vi "WaitForBufferExample.vi"() -> ()   [LabVIEW 2012]
doc: "A short program to demonstrate the fundamentals of control and image acquision with the pco.camera series. The program records a sequence of images, with \"live\" updating, until the \"StopRecording\" button is pressed. A subset of recorded images is then read out from the camera RAM. Warning: Limit the number of images read back tfrom the camera RAM to a reasonable number. Images are stored as a three-dimensional array, which can very large. Use ctrl-H for more help on the individual controls and indicators.\n\nCopyright 2004, the Cooke Corporation."
panel:
  out "bClose":bool
  in  "Quit":bool
  in  "ImageNr":i32
  in  "Image":i32
  out "BufNr1":i16
  out "BufNr0":i16
  in  "bUseBuffer1":bool
  in  "bUseBuffer0":bool
  in  "ROIX1":u16=1 min=1
  in  "ROIY1":u16=1 min=1
  in  "ROIY0":u16=1 min=1
  in  "ROIX0":u16=1 min=1
  in  "InterfaceType":u16(ring)=5 items=["IEEE1394 - Firewire", "IEEE1394/Firewire", "Matrox Helios Camera Link", "Silicon Software ME3 Camera Link", "National Instruments Camera Link", "Gigabit Ethernet", "USB", "Reserved", "Reserved", "Reserved", "Generic Camera Link with CLSER.DLL"]
  out "Bits/pixel":u16
  in  "Readout":bool
  in  "Record":bool
  in  "Open StructureIn":T1={"Size"=88, "InterfaceType"=0, "Camera Number"=0, "CameraNumAtInterface"=0, "OpenFlags"=[], "OpenDWFlags"=[], "OpenPtrs"=[]}
  in  "Stop":u32=10 min=1
  in  "Start":u32=1 min=1
  in  "DelayTimeBase":u16(ring)=2 items=["nanoseconds", "microseconds", "milliseconds"]
  in  "ExposureTimeBase":u16(ring)=2 items=["nanoseconds", "microseconds", "milliseconds"]
  in  "Exposure":u32=10
  in  "Delay":u32
  out "Reading":bool
  in  "StorageMode":bool
  out "ImageCount":u32
  in  "Rate":i32
  out "Image":u16[][](graph)
  in  "TriggerMode":u16(ring) items=["Auto", "Software", "External sequence start ", "External exposure control"]
  # "A short program to demonstrate the fundamentals of control and image acquision with the pco.camera series. The program records a sequence of images, with \"live\" updating, until the \"StopRecording\" button is pressed. A subset of recorded images is then read out from the camera RAM. WARNING: Limit the number of images read back tfrom the camera RAM to a reasonable number. Images are stored as a three-dimensional array, which can very large.  Use ctrl-H for more help on the individual controls and indicators."
  # "pco.labview"
  # "1) Setup camera:"
  # "FIFO"
  # "Recorder"
  # "2) Record  images:"
  # "3) Read out images:"
  # "4) Display image:"
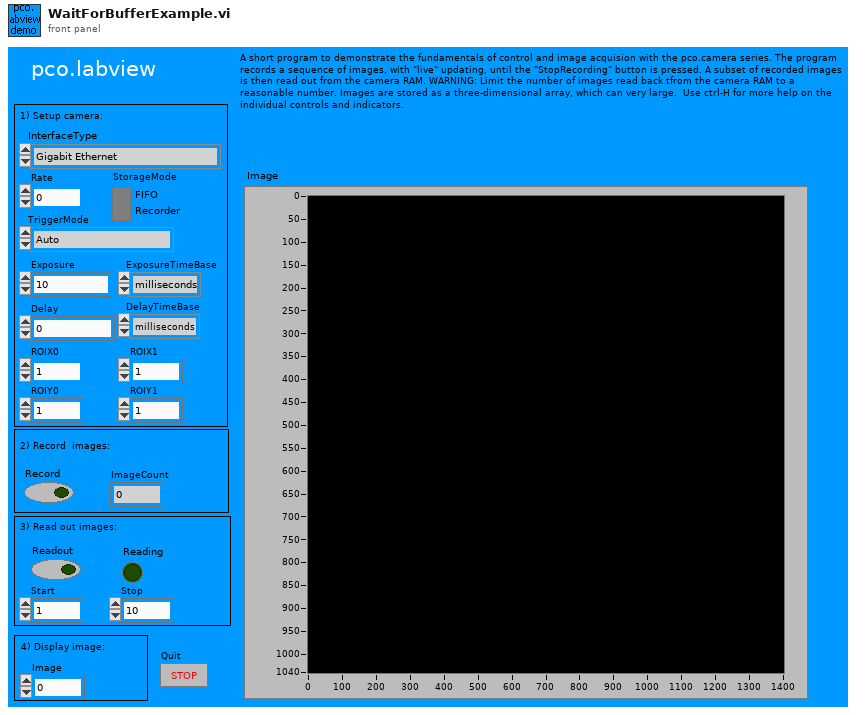
[diagram p1: front panel]
types:
  T1 = cluster{"Size":u16, "InterfaceType":u16, "Camera Number":u16, "CameraNumAtInterface":u16, "OpenFlags":u16[], "OpenDWFlags":u32[], "OpenPtrs":u32[]}
  T2 = cluster{"Size":u16, "CamType":u16, "CamSubType":u16, "SerialNumber":u32, "HWVersion":u32, "FWVersion":u32, "InterfaceType":u16, "HardwareVersion":cluster{"BoardNum":u16, "HWVersions":cluster{"BoardName":string, "BatchNumber":u16, "MinorRevision":u8, "MajorRevision":u8, "Variant":u16}[]}, "FirmwareVersion":cluster{"DeviceNum":u16, "FWVersions":cluster{"DeviceName":string, "MinorRevision":u8, "MajorRevision":u8, "Variant":u16}[]}}
  T3 = cluster{"Size":u16, "SensorTypeDESC":u16, "SensorSubtypeDESC":u16, "MaxHorizontalResStdDESC":u16, "MaxVerticalResStdDESC":u16, "MaxHorizontalResExtDESC":u16, "MaxVerticalResExtDESC":u16, "DynResDESC":u16, "MaxBinHorzDESC":u16, "BinHorzStepDESC":bool, "MaxBinVertDESC":u16, "BinVertStepDESC":bool, "ROIHorzStepDESC":u16, "ROIVertStepDESC":u16, "NumADCDESC":u16, "IRDESC":bool, "MinDelayDESC":u32, "MaxDelayDESC":u32, "MinDelayStepDESC":u32, "MinExpoDESC":u32, "MaxExpoDESC":u32, "MinExpoStepDESC":u32, "MinDelayIRDESC":u32, "MaxDelayIRDESC":u32, "MinExpoIRDESC":u32, "MaxExpoIRDESC":u32, "TimeTableDESC":bool, "DoubleImageDESC":bool, "MinCoolSetDESC":i16, "MaxCoolSetDESC":i16, "MDefaultCoolSetDESC":i16, "PowerDownModeDESC":bool, "OffsetRegDESC":bool, "ColorPattern":cluster{"UpperLeftColor":u8, "UpperRightColor":u8, "LowerLeftColor":u8, "LowerRightColor":u8}, "PatternTypeDESC":bool, "PixelRates":u32[], "CoversionFactors":u16[], "Reserved":u32[], "NoiseFilterCapable":bool, "HotPixelCapable":bool, "HotPixelWithNoiseFilter":bool, "ASCIITimeCapable":bool, "Extended Description":bool, "Get Extended":bool, "Reserved Flag 1":bool, "Reserved Flag 2":bool}
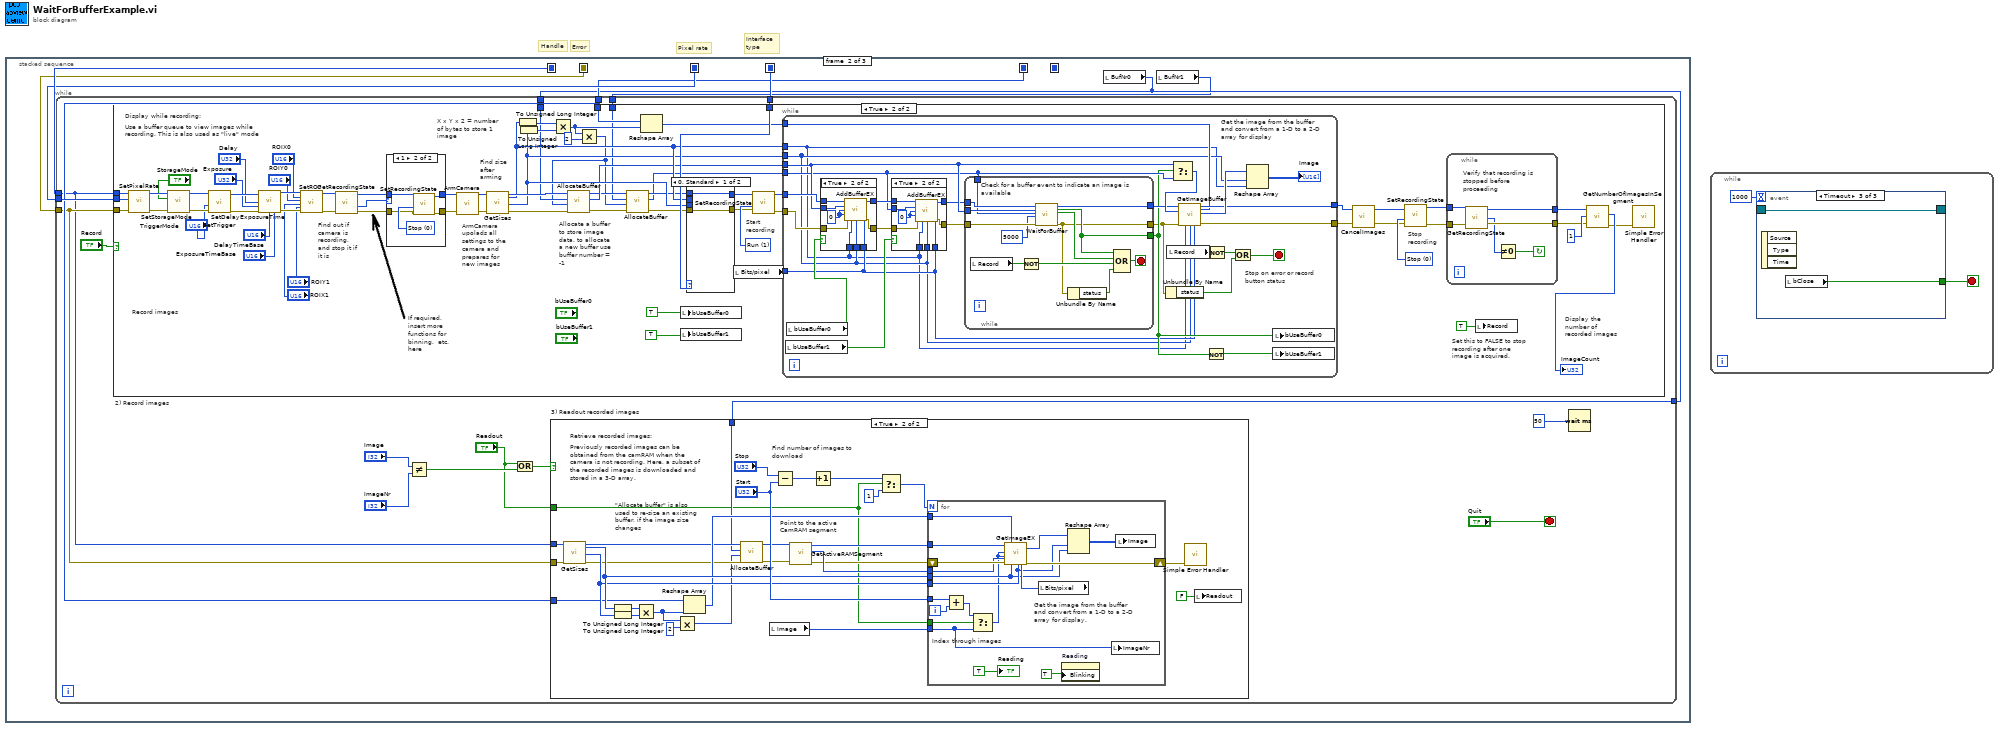
[diagram p0: block diagram]
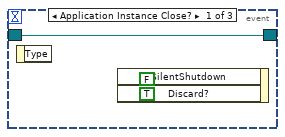
[diagram p2: hidden frame]
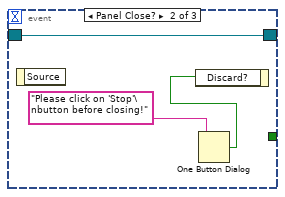
[diagram p3: hidden frame]
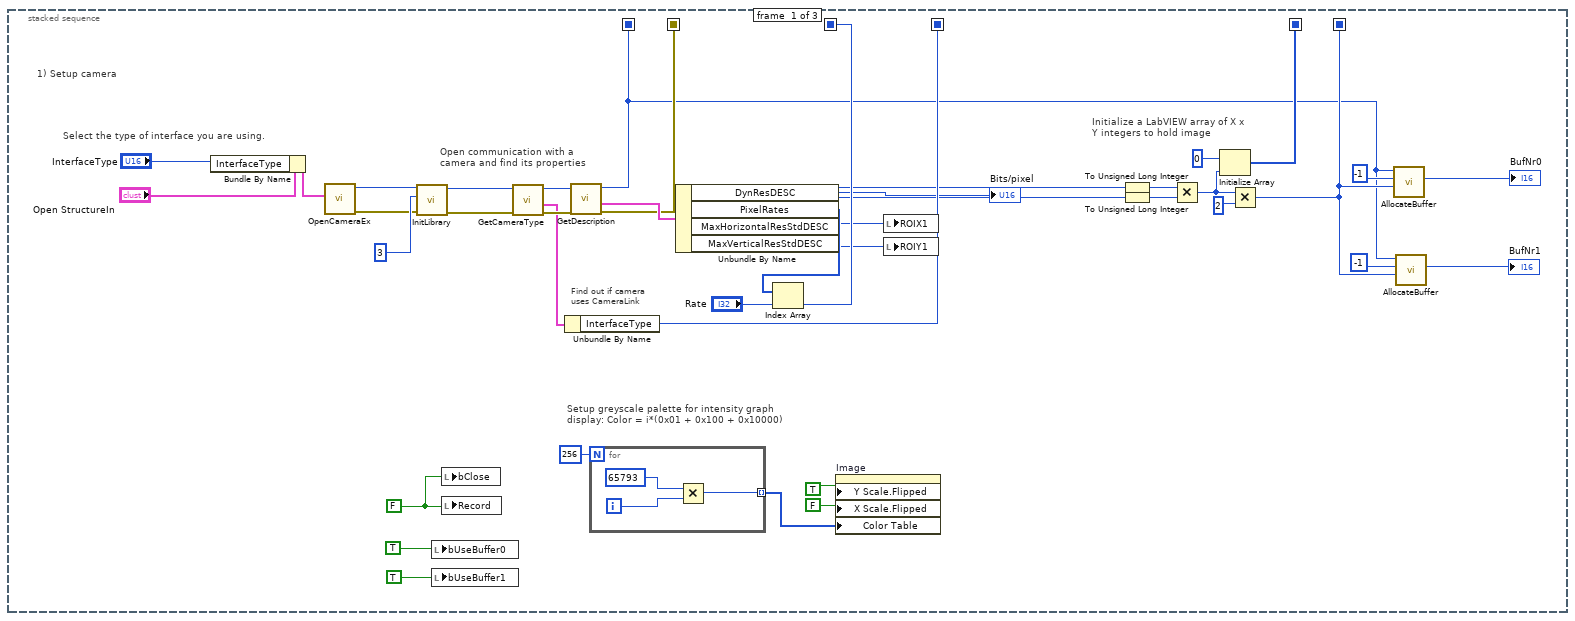
[diagram p4: hidden frame]
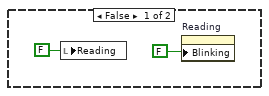
[diagram p5: hidden frame]
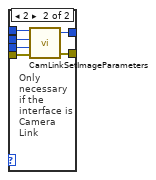
[diagram p9: hidden frame]
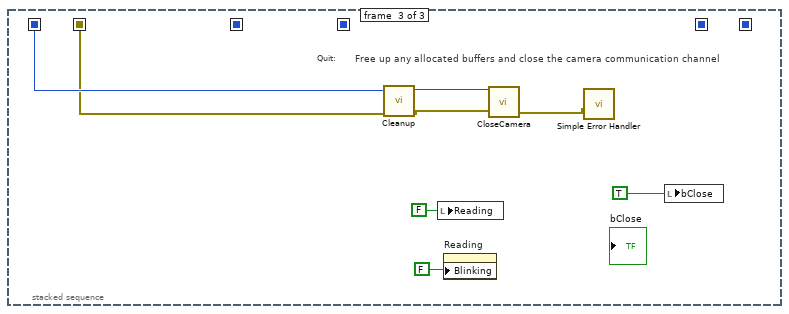
[diagram p11: hidden frame]
diagram:
  # "Interface type"
  # "Error"
  # "Handle"
  # "Pixel rate"
  n1 = stacked-sequence {
    seq-local: [w33 _ _] -> [_ w45 _]
    seq-local: [w13 _ _] -> [_ _ _]
    seq-local: [w25 _ _] -> [_ w47 _]
    seq-local: [w12 _ _] -> [_ w49 w270]
    seq-local: [w24 _ _] -> [_ w48 w269]
    seq-local: [w23 _ _] -> [_ w46 _]
    frame #0 {
      w6 = FALSE ("stop")
      # "Select the type of interface you are using."
      # "1) Setup camera"
      # "Find out if camera uses CameraLink"
      # "Setup greyscale palette for intensity graph display: Color = i*(0x01 + 0x100 + 0x10000)"
      # "Initialize a LabVIEW array of X x Y integers to hold image"
      # "Open communication with a camera and find its properties"
      n2 = Bundle By Name(cluster="Open StructureIn", "InterfaceType"="InterfaceType") -> (w20:T1)
      n3 = call "OpenCameraEx.vi"("OpenStructureIn"=w20) -> ("error out"=w3:errorcluster, "hout"=w4:u64)  [unwired: 3 in, 2 out]
      n4 = call "InitLibrary.vi"("error in (no error)"=w3, "InterfaceType"=u32 3, "ph"=w4) -> ("error out"=w1:errorcluster, "hout"=w2:u64)  [unwired: 7 in]
      n5 = local write "bUseBuffer0"(TRUE) -> ()
      n6 = local write "bUseBuffer1"(TRUE) -> ()
      n7 = local write "bClose"(w6) -> ()
      n8 = local write "Record"(w6) -> ()
      n9 = call "GetCameraType.vi"("ph"=w2, "error in (no error)"=w1) -> ("hout"=w29:u64, "CameraType"=w27:T2, "error out"=w28:errorcluster)  [unwired: 1 in, 1 out]
      n10 = Unbundle By Name(w27) -> ("InterfaceType"=w23:u16)
      n11 = call "GetDescription.vi"("ErrorIn"=w28, "ph"=w29) -> ("ErrorOut"=w24:errorcluster, "Description"=w32:T3, "hout"=w12:u64)  [unwired: 2 in, 1 out]
      n12 = for {
        N: 256 -> [_]
        tunnel: [w40] -> w36 mode=indexing
        i -> [w41]
        n13 = Multiply(x=65793, y=w41) -> (x*y=w40:i32)
      }
      n14 = Unbundle By Name(w32) -> ("DynResDESC"=→"Bits/pixel":u16, "PixelRates"=w26:u32[], "MaxHorizontalResStdDESC"=w18:u16, "MaxVerticalResStdDESC"=w17:u16)
      n15 = Index Array(array=w26, index="Rate") -> (element=w25:u32)
      n16 = property on="Image" class="IntGraph (strikt)"("Y Scale.Flipped"=TRUE, "X Scale.Flipped"=FALSE, "Color Table"=w36) -> ()  [unwired: 2 in, 2 out]
      n17 = local write "ROIX1"(w18) -> ()
      n18 = local write "ROIY1"(w17) -> ()
      n19 = To Unsigned Long Integer(number=w18) -> (unsigned 32bit integer=w15:u32)
      n20 = To Unsigned Long Integer(number=w17) -> (unsigned 32bit integer=w14:u32)
      n21 = Multiply(x=w15, y=w14) -> (x*y=w34:u32)
      n22 = Initialize Array(u16 0 ("Element Data"), w34) -> (w33:u16[])
      n23 = Multiply(x=w34, y=u32 2) -> (x*y=w13:u32)
      n24 = call "AllocateBuffer.vi"("Size"=w13, "BufNr"=i16 -1, "ph"=w12) -> ("BufNrOut"=→"BufNr0":i16)  [unwired: 3 in, 5 out]
      n25 = call "AllocateBuffer.vi"("Size"=w13, "BufNr"=-1, "ph"=w12) -> ("BufNrOut"=→"BufNr1":i16)  [unwired: 3 in, 5 out]
    }
    frame #1 {
      n26 = local read "BufNr0"() -> (w44:i16)
      n27 = local read "BufNr1"() -> (w43:i16)
      n28 = while {
        tunnel: w44 -> [w58]
        tunnel: w44 -> [w59]
        tunnel: w45 -> [w61]
        tunnel: w46 -> [w62]
        tunnel: w47 -> [w63]
        tunnel: w48 -> [w60]
        tunnel: w49 -> [w56]
        tunnel: w43 -> [w57]
        stop <- "Quit" stop-if-true
        n29 = case "2) Record images" shown="True" "Record" {
          tunnel: w56 -> [_ w158]
          tunnel: w60 -> [_ w157]
          tunnel: w63 -> [_ w155]
          tunnel: w62 -> [_ w154]
          tunnel: w61 -> [_ w152]
          tunnel: w59 -> [_ w135]
          tunnel: w57 -> [_ w129]
          frame False {
          }
          frame True {
            w182 = u16 1 items=["Stop", "Run"] ("RecordingState")
            w185 = u16 0 items=["Stop", "Run"] ("RecordingState")
            # "Set this to FALSE to stop recording after one image is acquired."
            # "Display the number of recorded images"
            # "Record images"
            # "Start recording"
            # "Allocate a buffer to store image data. to allocate a new buffer use buffer number = -1"
            # "Find size after arming"
            # "ArmCamera upolads all settings to the camera and prepares for new images"
            # "Find out if camera is recording, and stop it if it is"
            # "If required, insert more functions for binning.  etc. here"
            # "X x Y x 2 = number of bytes to store 1 image"
            # "Stop recording"
            # "Use a buffer queue to view images while recording. This is also used as \"live\" mode"
            # "Display while recording:"
            n30 = call "SetPixelRate.vi"("error in (no error)"=w157, "PixelRate"=w155, "ph"=w158) -> ("error out"=w180:errorcluster, "hout"=w181:u64)  [unwired: 2 in, 1 out]
            n31 = call "SetStorageMode.vi"("error in (no error)"=w180, "StorageMode"="StorageMode", "ph"=w181) -> ("error out"=w172:errorcluster, "hout"=w173:u64)  [unwired: 2 in, 1 out]
            n32 = call "SetTrigger.vi"("error in (no error)"=w172, "TriggerMode"="TriggerMode", "ph"=w173) -> ("error out"=w165:errorcluster, "hout"=w166:u64)  [unwired: 2 in, 1 out]
            n33 = call "SetDelayExposureTime.vi"("ph"=w166, "Delay"="Delay", "Exposure"="Exposure", "error in (no error)"=w165, "DelayTimeBase"="DelayTimeBase", "ExposureTimeBase"="ExposureTimeBase") -> ("hout"=w143:u64, "error out"=w141:errorcluster)  [unwired: 7 in, 1 out]
            n34 = call "SetROI.vi"("ph"=w143, "ROIX0"="ROIX0", "ROIY0"="ROIY0", "ROIX1"="ROIX1", "ROIY1"="ROIY1", "error in (no error)"=w141) -> ("hout"=w142:u64, "error out"=w140:errorcluster)  [unwired: 12 in]
            n35 = call "GetRecordingState.vi"("ErrorIn"=w140, "ph"=w142) -> ("ErrorOut"=w176:errorcluster, "RecordingState"=w178:u16, "hout"=w177:u64)  [unwired: 2 in, 1 out]
            n36 = case shown="1" w178 {
              tunnel: w177 -> [w263 w267]
              tunnel: w176 -> [w262 w266]
              tunnel: [w263 w265] -> w175
              tunnel: [w262 w264] -> w174
              frame 0, Default {
              }
              frame 1 {
                w268 = u16 0 items=["Stop", "Run"] ("RecordingState")
                n37 = call "SetRecordingState.vi"("ErrorIn"=w266, "RecordingState"=w268, "ph"=w267) -> ("ErrorOut"=w264:errorcluster, "hout"=w265:u64)  [unwired: 2 in, 1 out]
              }
            }
            n38 = call "ArmCamera.vi"("error in (no error)"=w174, "ph"=w175) -> ("error out"=w170:errorcluster, "hout"=w171:u64)  [unwired: 1 in, 1 out]
            n39 = call "GetSizes.vi"("ph"=w171, "ErrorIn"=w170) -> ("hout"=w167:u64, "XResAct"=w150:u16, "YResAct"=w149:u16, "ErrorOut"=w169:errorcluster)  [unwired: 11 in, 3 out]
            n40 = To Unsigned Long Integer(number=w150) -> (unsigned 32bit integer=w144:u32)
            n41 = To Unsigned Long Integer(number=w149) -> (unsigned 32bit integer=w145:u32)
            n42 = Multiply(x=w144, y=w145) -> (x*y=w146:u32)
            n43 = Multiply(x=w146, y=u32 2) -> (x*y=w130:u32)
            n44 = call "AllocateBuffer.vi"("error in (no error)"=w169, "Size"=w130, "BufNr"=w135, "ph"=w167) -> ("error out"=w134:errorcluster, "BufNrOut"=w147:i16, "hout"=w132:u64)  [unwired: 2 in, 3 out]
            n45 = call "AllocateBuffer.vi"("error in (no error)"=w134, "Size"=w130, "BufNr"=w129, "ph"=w132) -> ("error out"=w133:errorcluster, "BufNrOut"=w128:i16, "hout"=w131:u64)  [unwired: 2 in, 3 out]
            n46 = Reshape Array(w152, w146) -> (w151:u16[])
            n47 = local write "bUseBuffer0"(TRUE) -> ()
            n48 = local write "bUseBuffer1"(TRUE) -> ()
            n49 = case shown="0, Standard" w154 {
              tunnel: w133 -> [w254 w261]
              tunnel: [w254 w260] -> w160
              tunnel: w131 -> [w255 w259]
              tunnel: [w255 w258] -> w159
              tunnel: w149 -> [_ w257]
              tunnel: w150 -> [_ w256]
              frame 0, Default {
              }
              frame 2 {
                # "Only necessary if the interface is Camera Link"
                n50 = call "CamLinkSetImageParameters.vi"("error in (no error)"=w261, "YRes"=w257, "XRes"=w256, "ph"=w259) -> ("error out"=w260:errorcluster, "hout"=w258:u64)  [unwired: 1 out]
              }
            }
            n51 = local read "Bits/pixel"() -> (w121:u16)
            n52 = call "SetRecordingState.vi"("ErrorIn"=w160, "RecordingState"=w182, "ph"=w159) -> ("ErrorOut"=w156:errorcluster, "hout"=w153:u64)  [unwired: 2 in, 1 out]
            n53 = while {
              tunnel: w147 -> [w198]
              tunnel: w151 -> [w208]
              tunnel: w153 -> [w207]
              tunnel: w149 -> [w187]
              tunnel: w150 -> [w186]
              tunnel: w156 -> [w205]
              tunnel: [w210] -> w120
              tunnel: [w211] -> w119
              tunnel: w128 -> [w197]
              tunnel: w121 -> [w188]
              stop <- w189 stop-if-true
              # "Stop on error or record button status"
              # "Get the image from the buffer and convert from a 1-D to a 2-D array for display"
              n54 = local read "bUseBuffer1"() -> (w202:bool)
              n55 = local read "bUseBuffer0"() -> (w203:bool)
              n56 = case shown="True" w203 {
                tunnel: [w214 w223] -> w204
                tunnel: [w213 w222] -> w206
                tunnel: w198 -> [_ w221]
                tunnel: w207 -> [w213 w220]
                tunnel: w188 -> [_ w218]
                tunnel: w186 -> [_ w217]
                tunnel: w187 -> [_ w216]
                tunnel: w205 -> [w214 w215]
                frame False {
                }
                frame True {
                  w219 = 0
                  n57 = call "AddBufferEX.vi"("ph"=w220, "BuffNr"=w221, "1stImage"=w219, "LastImage"=w219, "error in (no error)"=w215, "XRes"=w217, "YRes"=w216, "BitPerPixel"=w218) -> ("hout"=w222:u64, "error out"=w223:errorcluster)  [unwired: 5 in, 1 out]
                }
              }
              n58 = case shown="True" w202 {
                tunnel: [w224 w234] -> w195
                tunnel: [w225 w233] -> w196
                tunnel: w197 -> [_ w232]
                tunnel: w206 -> [w225 w231]
                tunnel: w188 -> [_ w229]
                tunnel: w186 -> [_ w228]
                tunnel: w187 -> [_ w227]
                tunnel: w204 -> [w224 w226]
                frame False {
                }
                frame True {
                  w230 = 0
                  n59 = call "AddBufferEX.vi"("ph"=w231, "BuffNr"=w232, "1stImage"=w230, "LastImage"=w230, "error in (no error)"=w226, "XRes"=w228, "YRes"=w227, "BitPerPixel"=w229) -> ("hout"=w233:u64, "error out"=w234:errorcluster)  [unwired: 5 in, 1 out]
                }
              }
              n60 = while {
                tunnel: w198 -> [w242]
                tunnel: w197 -> [w241]
                tunnel: w196 -> [w244]
                tunnel: w195 -> [w243]
                tunnel: [w240] -> w194
                tunnel: [w236] -> w192
                tunnel: [w239] -> w193
                stop <- w245 stop-if-true
                # "Check for a buffer event to indicate an image is available"
                n61 = local read "Record"() -> (w247:bool)
                n62 = Not(x=w247) -> (.not. x?=w246:bool)
                n63 = call "WaitForBuffer.vi"("ph"=w244, "sBufNr"=w242, "sBufNr 2"=w241, "timeout"=5000, "error in (no error)"=w243) -> ("hout"=w240:u64, "Buffer_Ready"=w239:bool, "Buffer_Ready 2"=w238:bool, "error out"=w236:errorcluster)  [unwired: 10 in, 1 out]
                n64 = Unbundle By Name(w236) -> ("status"=w235:bool)
                n65 = Compound Arithmetic op=OR(w239, w238, w246, w235) -> (w245:bool)
              }
              n66 = Unbundle By Name(w192) -> ("status"=w190:bool)
              n67 = local read "Record"() -> (w209:bool)
              n68 = Select(t=w198, s=w193, f=w197) -> (s? t:f=w201:i16)
              n69 = call "GetImageBuffer.vi"("ph"=w194, "BuffIn"=w208, "BuffNr"=w201, "error in (no error)"=w192, "xRes"=w186, "yRes"=w187, "Bitresolution"=w188) -> ("hout"=w210:u64, "BuffOut"=w212:u16[], "error out"=w211:errorcluster)  [unwired: 5 in, 1 out]
              n70 = Not(x=w193) -> (.not. x?=w200:bool)
              n71 = Not(x=w209) -> (.not. x?=w191:bool)
              n72 = Or(x=w191, y=w190) -> (x .or. y?=w189:bool)
              n73 = Reshape Array(w212, w187, w186) -> (→"Image":u16[][])
              n74 = local write "bUseBuffer0"(w193) -> ()
              n75 = local write "bUseBuffer1"(w200) -> ()
            }
            n76 = call "CancelImages.vi"("error in (no error)"=w119, "ph"=w120) -> ("error out"=w125:errorcluster, "hout"=w124:u64)  [unwired: 1 in, 1 out]
            n77 = call "SetRecordingState.vi"("ErrorIn"=w125, "RecordingState"=w185, "ph"=w124) -> ("ErrorOut"=w183:errorcluster, "hout"=w184:u64)  [unwired: 2 in, 1 out]
            n78 = while {
              tunnel: [w251] -> w118
              tunnel: w183 -> [w252]
              tunnel: w184 -> [w253]
              tunnel: [w248] -> w117
              stop <- w249 continue-if-true
              # "Verify that recording is stopped before proceeding"
              n79 = call "GetRecordingState.vi"("ErrorIn"=w252, "ph"=w253) -> ("ErrorOut"=w251:errorcluster, "RecordingState"=w250:u16, "hout"=w248:u64)  [unwired: 2 in, 1 out]
              n80 = Not Equal To 0?(x=w250) -> (x != 0?=w249:bool)
            }
            n81 = local write "Record"(TRUE ("Record")) -> ()
            n82 = call "GetNumberOfImagesInSegment.vi"("ph"=w117, "Segment"=u16 1, "error in (no error)"=w118) -> ("ValidImageCnt"=→"ImageCount":u32, "error out"=w116:errorcluster)  [unwired: 3 out]
            n83 = call <vilib>:"Simple Error Handler.vi"("error in (no error)"=w116) -> ()  [unwired: 4 in, 5 out]
          }
        }
        n84 = Not Equal?(x="Image", y="ImageNr") -> (x != y?=w53:bool)
        n85 = Or(x="Readout", y=w53) -> (x .or. y?=w52:bool)
        n86 = case "3) Readout recorded images" shown="True" w52 {
          tunnel: w61 -> [_ w89]
          tunnel: w56 -> [_ w81]
          tunnel: w60 -> [_ w80]
          tunnel: w58 -> [_ w74]
          tunnel: "Readout" -> [_ w68]
          frame False {
            n87 = local write "Reading"(FALSE ("Reading")) -> ()
            n88 = property on="Reading" class="Bool. (strikt)"("Blinking"=FALSE) -> ()  [unwired: 2 in, 2 out]
          }
          frame True {
            # "Point to the active CamRAM segment"
            # "\"Allocate buffer\" is also used to re-size an existing buffer, if the image size changes"
            # "Find number of images to download"
            # "Previously recorded images can be obtained from the camRAM when the camera is not recording. Here, a subset of the recorded images is downloaded and stored in a 3-D array."
            # "Retrieve recorded images:"
            n89 = call "GetSizes.vi"("ph"=w81, "ErrorIn"=w80) -> ("hout"=w87:u64, "XResAct"=w91:u16, "YResAct"=w90:u16, "ErrorOut"=w85:errorcluster)  [unwired: 11 in, 3 out]
            n90 = To Unsigned Long Integer(number=w91) -> (unsigned 32bit integer=w77:u32)
            n91 = To Unsigned Long Integer(number=w90) -> (unsigned 32bit integer=w78:u32)
            n92 = Multiply(x=w77, y=w78) -> (x*y=w79:u32)
            n93 = Multiply(x=w79, y=u32 2) -> (x*y=w76:u32)
            n94 = Reshape Array(w89, w79) -> (w88:u16[])
            n95 = call "AllocateBuffer.vi"("error in (no error)"=w85, "Size"=w76, "BufNr"=w74, "ph"=w87) -> ("error out"=w84:errorcluster, "hout"=w86:u64)  [unwired: 2 in, 4 out]
            n96 = local read "Image"() -> (w72:i32)
            n97 = Subtract(x="Stop", y="Start") -> (x-y=w95:u32)
            n98 = call "GetActiveRAMSegment.vi"("error in (no error)"=w84, "ph"=w86) -> ("error out"=w82:errorcluster, "ActSeg"=w92:u16, "hout"=w83:u64)  [unwired: 2 in, 1 out]
            n99 = Increment(x=w95) -> (x+1=w71:u32)
            n100 = Select(t=w71, s=w68, f=1) -> (s? t:f=w70:u32)
            n101 = for {
              N: w70 -> [_]
              tunnel: w83 -> [w114]
              shift-right: [w111] -> w73
              shift-left: w82 -> [w110]
              tunnel: "Start" -> [w107]
              tunnel: w92 -> [w105]
              tunnel: w91 -> [w101]
              tunnel: w90 -> [w102]
              tunnel: w88 -> [w103]
              tunnel: w72 -> [w97]
              tunnel: w68 -> [w99]
              i -> [w106]
              # "Get the image from the buffer and convert from a 1-D to a 2-D array for display."
              # "Index through images"
              n102 = Add(x=w107, y=w106) -> (x+y=w98:u32)
              n103 = Select(t=w98, s=w99, f=w97) -> (s? t:f=w100:u32)
              n104 = local read "Bits/pixel"() -> (w104:u16)
              n105 = call "GetImageEX.vi"("ph"=w114, "1stImage"=w100, "lastImage"=w100, "segment"=w105, "error in (no error)"=w110, "BuffIn"=w103, "xRes"=w101, "yRes"=w102, "BitPerPixel"=w104) -> ("BuffOut"=w113:u16[], "error out"=w111:errorcluster)  [unwired: 7 in, 2 out]
              n106 = property on="Reading" class="Bool. (strikt)"("Blinking"=TRUE) -> ()  [unwired: 2 in, 2 out]
              n107 = Reshape Array(w113, w102, w101) -> (w112:u16[][])
              n108 = local write "ImageNr"(w97) -> ()
              n109 = local write "Image"(w112) -> ()
              "Reading" <- TRUE ("Reading")
            }
            n110 = call <vilib>:"Simple Error Handler.vi"("error in (no error)"=w73) -> ()  [unwired: 4 in, 5 out]
            n111 = local write "Readout"(FALSE ("Readout")) -> ()
          }
        }
        n112 = Wait (ms)(milliseconds to wait=u32 50) -> ()  [unwired: 1 out]
      }
    }
    frame #2 {
      # "Free up any allocated buffers and close the camera communication channel"
      # "Quit:"
      n113 = call "Cleanup.vi"("error in (no error)"=w269, "ph"=w270) -> ("error out"=w272:errorcluster, "hout"=w271:u64)  [unwired: 8 in]
      n114 = local write "Reading"(FALSE ("Reading")) -> ()
      n115 = property on="Reading" class="Bool. (strikt)"("Blinking"=FALSE) -> ()  [unwired: 2 in, 2 out]
      n116 = call "CloseCamera.vi"("ErrorIn"=w272, "Handle in"=w271) -> ("ErrorOut"=w274:errorcluster)  [unwired: 1 in, 2 out]
      n117 = call <vilib>:"Simple Error Handler.vi"("error in (no error)"=w274) -> ()  [unwired: 4 in, 5 out]
      n118 = local write "bClose"(TRUE) -> ()
    }
  }
  n119 = while {
    stop <- w277 stop-if-true
    n120 = event shown="[2] Timeout" {
      selector: _ -> [w279 w284 w286]
      dyn-events: [w279 w284 w286] -> _
      timeout: 1000 -> [_ _ _]
      tunnel: [_ _ w285] -> w277
      event Application Instance Close? {
        n121 = event-data() -> ()  [unwired: 1 in, 1 out]
        n122 = event-data("SilentShutdown"=FALSE, "Discard?"=TRUE) -> ()  [unwired: 1 in, 1 out]
      }
      event Panel Close? {
        n123 = event-data() -> ()  [unwired: 1 in, 1 out]
        n124 = One Button Dialog(message="Please click on 'Stop'\nbutton before closing!") -> (true=w282:bool)  [unwired: 1 in]
        n125 = event-data("Discard?"=w282) -> ()  [unwired: 1 in, 1 out]
      }
      event Timeout {
        n126 = event-data() -> ()  [unwired: 1 in, 3 out]
        n127 = local read "bClose"() -> (w285:bool)
      }
    }
  }
